vi "is image clear.vi"(0 "Input image":T1) -> (1 "Image Out":T1, 2 "Image ok":bool, 3 "error out":errorcluster)   [LabVIEW 2013]
uses:
  <vilib>/vision/Image Controls.llb/IMAQ Image.ctl
  <vilib>/vision/NI_Vision_Development_Module.lvlib
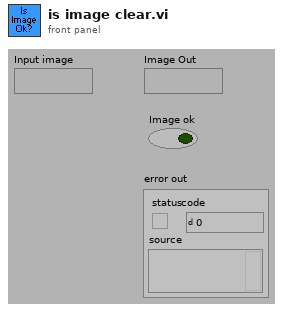
[diagram p1: front panel]
types:
  T1 = typedef "IMAQ Image.ctl" = refnum<image>
  T2 = typedef "IMAQ Rectangle" = cluster{"Left":i32, "Top":i32, "Right":i32, "Bottom":i32, "Rotation":dbl}
  T3 = cluster{"Mean Intensity":sgl, "Standard  Deviation":sgl, "Minimum Intensity":sgl, "Maximum Intensity":sgl}
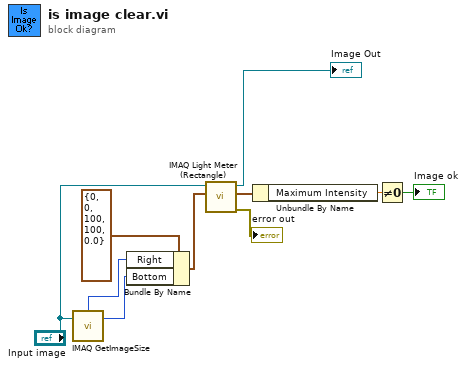
[diagram p0: block diagram]
diagram:
  n1 = call "IMAQ GetImageSize"("Image"="Input image") -> ("Y Resolution"=w8:i32, "X Resolution"=w7:i32)  [unwired: 3 in, 1 out]
  n2 = Bundle By Name(cluster=T2 {"Left"=0, "Top"=0, "Right"=100, "Bottom"=100, "Rotation"=0.0} ("Rectangle"), "Right"=w7, "Bottom"=w8) -> (w6:T2)
  n3 = call "IMAQ Light Meter (Rectangle)"("Rectangle"=w6, "Image"="Input image") -> ("error out"=→"error out":errorcluster, "Gray Level Intensities"=w3:T3, "Image Out"=→"Image Out":T1)  [unwired: 5 in, 2 out]
  n4 = Unbundle By Name(w3) -> ("Maximum Intensity"=w2:sgl)
  n5 = Not Equal To 0?(x=w2) -> (x != 0?=→"Image ok":bool)
